vi "Main.vi"() -> ()   [LabVIEW 2010]
uses:
  <vilib>/Instr/_visa.llb/VISA Set IO Buffer Mask.ctl
  <vilib>/Instr/_visa.llb/VISA Flush IO Buffer Mask.ctl
  GlobalVar.vi
  <vilib>/Instr/_visa.llb/VISA Configure Serial Port (Instr).vi
panel:
  out "Frequency":dbl
  out "Enum":T1(ring)
  out "error":errorcluster
  out "error Connexion":errorcluster
  out "Stop main loop":bool
  in  "stop":bool
  in  "Tab Control":T2(tab)
  out "Comm_LEDTest":bool
  out "Comm_Reception":string caption="Reception"
  in  "Comm_TestConnection":bool
  in  "Comm_BaudRate":u32=9600 caption="Baud rate"
  in  "Comm_PortComm":refnum<visa-resource-name>="COM7" caption="Communication Port"
  in  "timeout (10sec)":u32=10000
  in  "Con_RefreshIntensity":bool caption="Bouton OK 12"
  in  "Con_RefreshRightTorque":bool caption="Bouton OK 12"
  out "Con_XYIntensity":cluster{"Y":dbl[], "Y":dbl[]}[](graph) caption="Intensity"
  out "Con_XYRightTorque":cluster{"Y":dbl[], "Y":dbl[]}[](graph) caption="Motor right Torque"
  in  "Con_RefreshLeftTorque":bool caption="Bouton OK 12"
  out "Con_XYLeftTorque":cluster{"Y":dbl[], "Y":dbl[]}[](graph) caption="Motor left Torque"
  out "Con_IntensityMax":bool caption="Max Intensity"
  in  "Con_Intensity":string[][](array[string]) caption="Intensity (A)"
  in  "Con_MotorRightTorque":string[][](array[string]) caption="Motor right Torque (N.m)"
  out "Con_MotorLeftTorque":string[][](array[string]) caption="Motor left Torque (N.m)"
  in  "Ana_RefreshBattery":bool caption="Bouton OK 12"
  out "Ana_XYBattery":cluster{"Y":dbl[], "Y":dbl[]}[](graph) caption="Motor left Torque"
  in  "Ana_RefreshHandlebar":bool caption="Bouton OK 12"
  out "Ana_XYHandlebar":cluster{"Y":dbl[], "Y":dbl[]}[](graph) caption="Motor left Torque"
  out "Ana_Battery":string[][](array[string]) caption="Battery"
  out "Ana_Handlebar":string[][](array[string]) caption="Handlebar"
  in  "Inc_RefreshAcceleration":bool caption="Bouton OK 12"
  out "Ana_XYHandlebar 4":cluster{"Y":dbl[], "Y":dbl[]}[](graph) caption="Motor left Torque"
  in  "Inc_RefreshVelocityRightMotor":bool caption="Bouton OK 12"
  out "Ana_XYHandlebar 3":cluster{"Y":dbl[], "Y":dbl[]}[](graph) caption="Motor left Torque"
  in  "Inc_RefreshVelocityLeftMotor":bool caption="Bouton OK 12"
  out "Ana_XYHandlebar 2":cluster{"Y":dbl[], "Y":dbl[]}[](graph) caption="Motor left Torque"
  out "Inc_Acceleration":string[][](array[string]) caption="Acceleration"
  out "Inc_VelocityRightMotor":string[][](array[string]) caption="Velocity Right motor"
  out "Inc_VelocityLeftMotor":string[][](array[string]) caption="Velocity left motor"
  out "Other_AngleOUT":string[][](array[string]) caption="Angle Out of range"
  out "Other_SpeedSaturation":string[][](array[string]) caption="Speed saturation"
  out "Other_Distance":string[][](array[string]) caption="Distance"
  out "Other_Angle":string[][](array[string]) caption="Angle"
  out "Spe_XY":cluster{dbl, dbl}[](graph) caption="XY Graph"
  in  "Spe_Time":dbl caption="Time"
  in  "Spe_SendAnalysis":bool caption="Send Analysis"
  in  "Spe_Frequency":dbl caption="Frequency"
  in  "Spe_Liste":string(combo) caption="Type"
  in  "Config_VelocitySaturation":dbl caption="VelocitySaturation"
  in  "Config_Sendvelocitysaturation":bool caption="Set velocity saturation"
  out "Config_Ready":string caption="Ready"
  out "Config_CurrentState":string caption="Current state"
  in  "Config_SendReady":bool caption="Ready ?"
  in  "Config_SendCurrentState":bool caption="Current state ?"
  in  "Config_SendRestart":bool caption="Re Start system"
  in  "Config_SendSTOP":bool caption="STOP system"
  out "Config_tCoefKalman":dbl caption="tCoef Kalman"
  in  "Config_ReceiveKalman":bool
  in  "Config_SendCoefKalman":bool
  in  "Config_CoefKalman":dbl caption="Coef Kalman"
  in  "Config_SendCoefAcc":bool
  in  "Config_CoefAcc":dbl caption="Coef System Acc"
  out "Config_Coefdir":dbl caption="tCoef direction"
  in  "Config_SendCoefDir":bool
  in  "Coef DIR":dbl
  in  "Config_ReceiveCoefDir":bool
  out "Config_tD":dbl caption="tD"
  out "Config_tI":dbl caption="tI"
  out "Config_tK":dbl caption="tK"
  in  "Config_ReceiveD":bool caption="Bouton OK 6"
  in  "Config_ReceiveI":bool
  in  "Config_ReceiveK":bool
  in  "Config_SendD":bool
  in  "Config_SendI":bool
  in  "Config_SendK":bool
  in  "Config_D":dbl caption="D"
  in  "Config_I":dbl caption="I"
  in  "Config_K":dbl caption="K"
  in  "Config_SendPID":bool
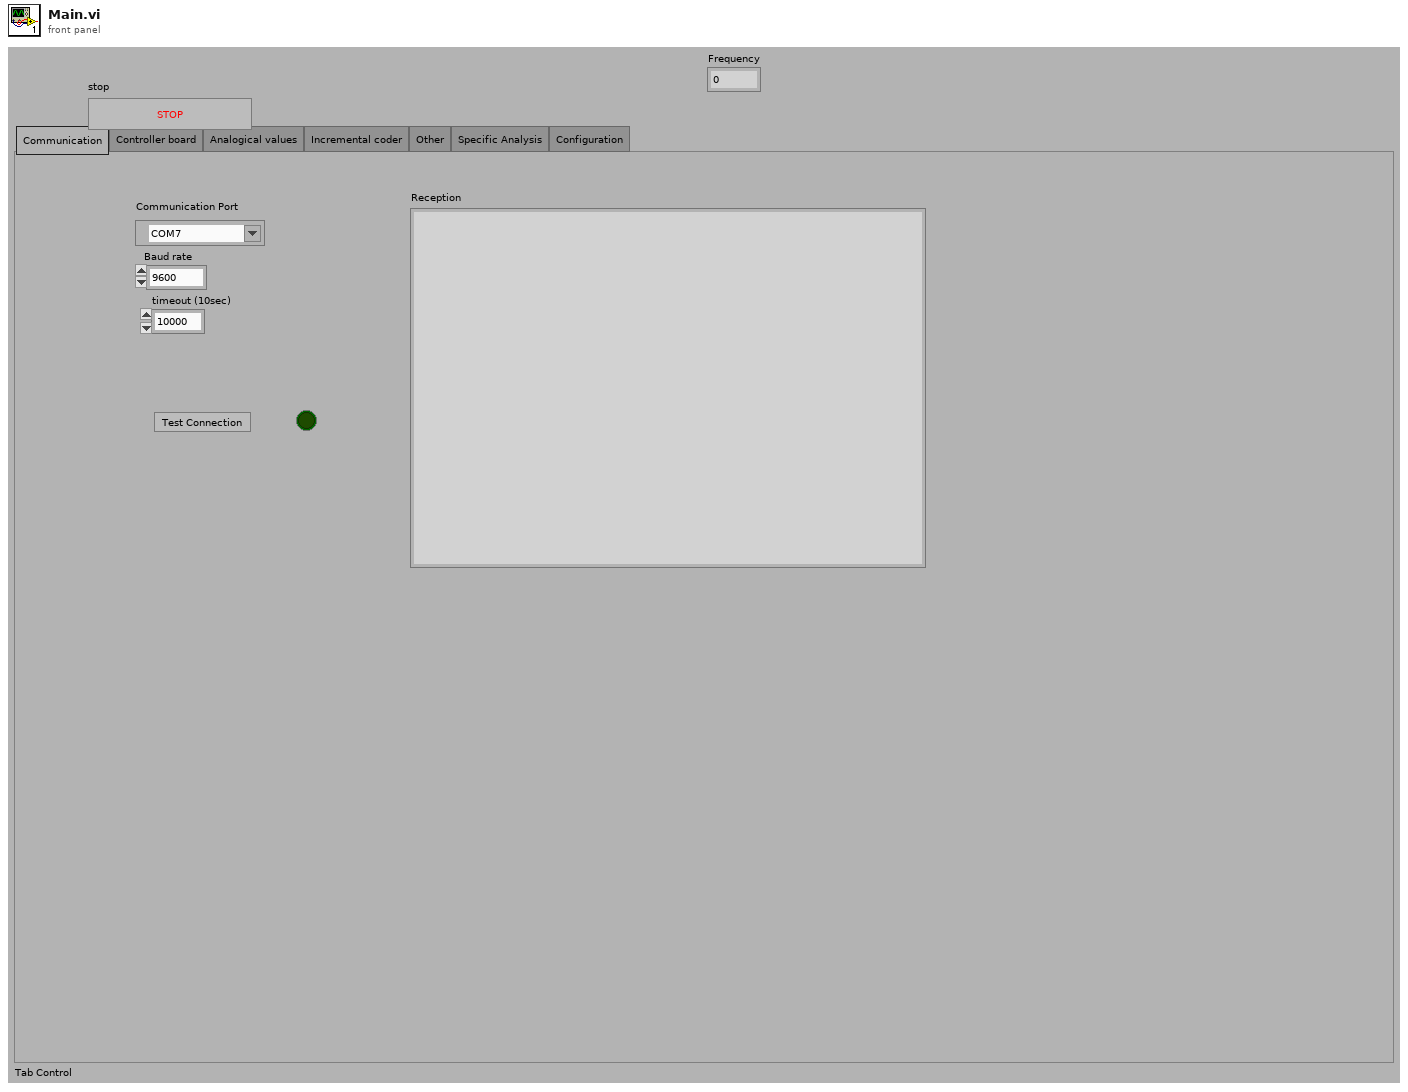
[diagram p1: front panel]
types:
  T1 = enum16{"SendAnalysis", "TestConnection", "Waiting"}
  T2 = enum32{"Communication", "Controller board", "Analogical values", "Incremental coder", "Other", "Specific Analysis", "Configuration"}
  T3 = typedef "VISA Set IO Buffer Mask.ctl" = u16
  T4 = typedef "VISA Flush IO Buffer Mask.ctl" = u16
  T5 = enum8{"Enabled", "Disabled", "Disabled and Grayed Out"}
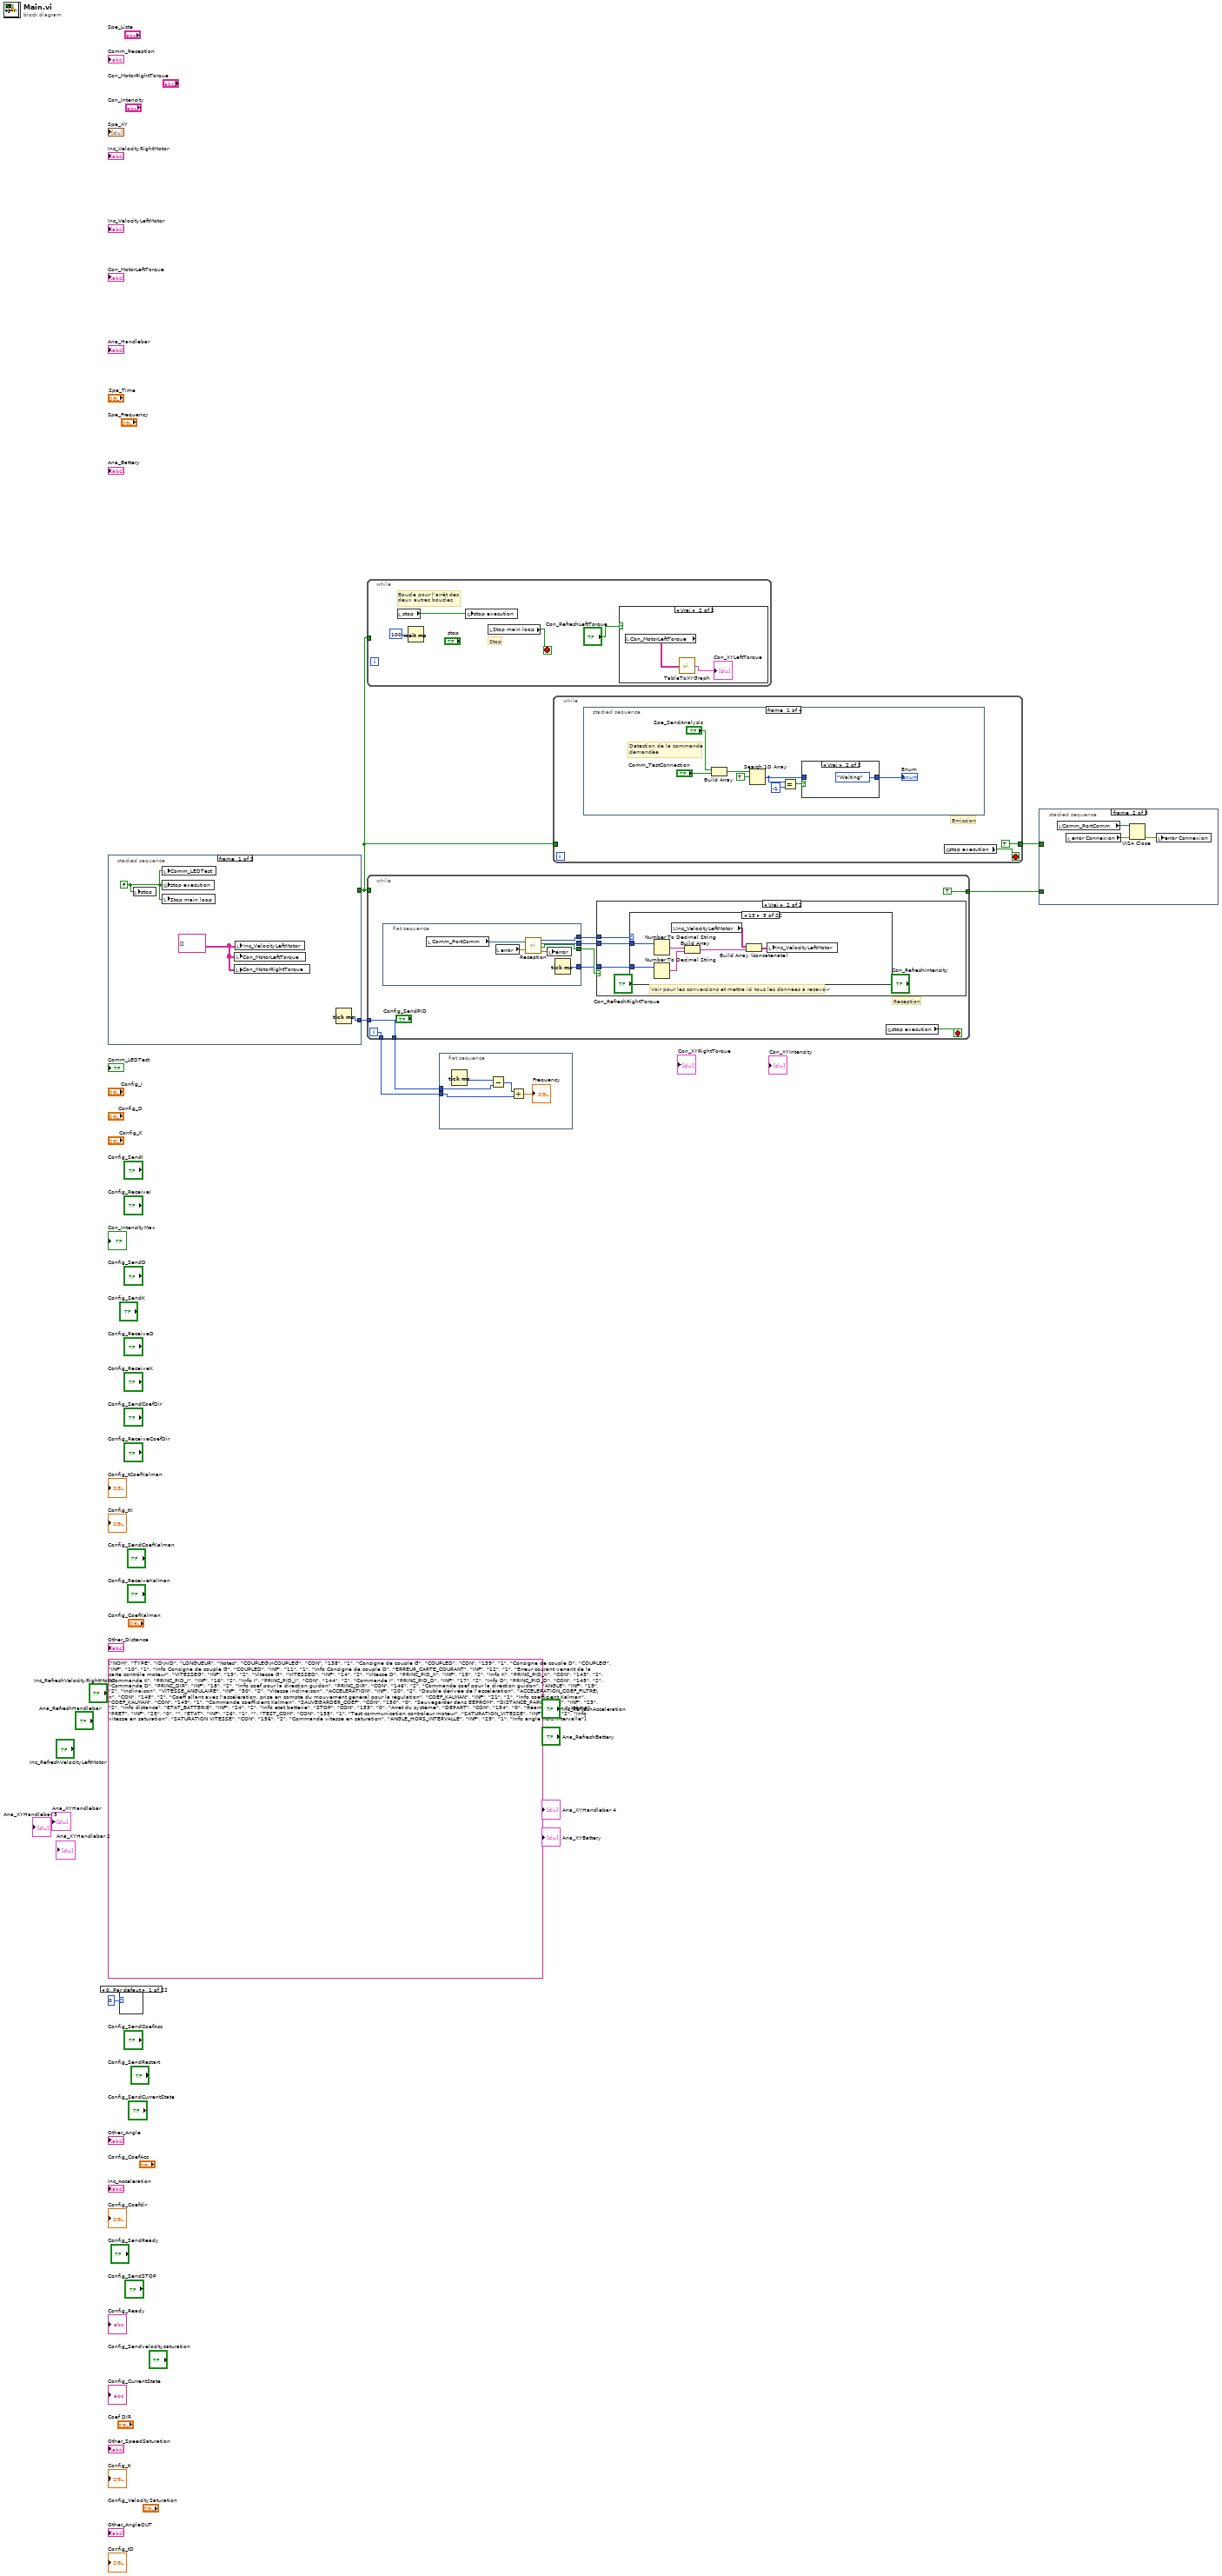
[diagram p0: block diagram]
diagram:
  (unwired) string[][] [["NOM", "TYPE", "ID\nID", "LONGUEUR", "Notes"], ["COUPLEG\nCOUPLEG", "CON", "138", "1", "Consigne de couple G"], ["COUPLED", "CON", "139", "1", "Consigne de couple D"], ["COUPLEG", "INF", "10", "1", "Info Consigne de couple G"], ["COUPLED", "INF", "11", "1", "Info Consigne de couple D"], ["ERREUR_CARTE_COURANT", "INF", "12", "1", "Erreur courant venant de la carte contrôle moteur"], ["VITESSEG", "INF", "13", "2", "Vitesse G"], ["VITESSED", "INF", "14", "2", "Vitesse D"], ["PRINC_PID_K", "INF", "15", "2", "Info K"], ["PRINC_PID_K", "CON", "143", "2", "Commande K"], ["PRINC_PID_I", "INF", "16", "2", "Info I"], ["PRINC_PID_I", "CON", "144", "2", "Commande I"], ["PRINC_PID_D", "INF", "17", "2", "Info D"], ["PRINC_PID_D", "CON", "145", "2", "Commande D"], ["PRINC_DIR", "INF", "18", "2", "Info coef pour la direction guidon"], ["PRINC_DIR", "CON", "146", "2", "Commande coef pour la direction guidon"], ["ANGLE", "INF", "19", "2", "Inclinaison"], ["VITESSE_ANGULAIRE", "INF", "30", "2", "Vitesse inclinaison"], ["ACCELERATION", "INF", "20", "2", "Double dérivée de l'accélération"], ["ACCELERATION_COEF_FILTRE\n", "CON", "148", "2", "Coeff allant avec l'accélération, prise en compte du mouvement général pour la régulation"], ["COEF_KALMAN", "INF", "21", "1", "Info coefficient Kalman"], ["COEF_KALMAN", "CON", "149", "1", "Commande coefficient Kalman"], ["SAUVEGARDER_COEF", "CON", "150", "0", "Sauvegarder dans EEPROM"], ["DISTANCE_PARCOURUE", "INF", "23", "2", "Info distance"], ["ETAT_BATTERIE", "INF", "24", "2", "Info etat batterie"], ["STOP", "CON", "153", "0", "Arret du système"], ["DEPART", "CON", "154", "0", "Réarmage du système"], ["PRET", "INF", "25", "0", ""], ["ETAT", "INF", "26", "1", ""], ["TEST_COM", "CON", "155", "1", "Test communication controleur moteur"], ["SATURATION_VITESSE", "INF", "28", "2", "Info vitesse en saturation"], ["SATURATION VITESSE", "CON", "156", "2", "Commande vitesse en saturation"], ["ANGLE_HORS_INTERVALLE", "INF", "29", "1", "Info angle hors intervalle"]]
  n1 = stacked-sequence {
    tunnel: [_ _ TRUE] -> w7
    tunnel: [w8 _ _] -> w3
    frame #0 {
      w9 = string[][] [] ("Velocity motor left")
      w10 = FALSE ("Comm_LEDTest")
      n2 = local write "stop"(w10) -> ()
      n3 = local write "Comm_LEDTest"(w10) -> ()
      n4 = global write "GlobalVar.vi" "stop execution"(w10) -> ()
      n5 = local write "Stop main loop"(w10) -> ()
      n6 = local write "Con_MotorLeftTorque"(w9) -> ()
      n7 = local write "Con_MotorRightTorque"(w9) -> ()
      n8 = local write "Inc_VelocityLeftMotor"(w9) -> ()
      n9 = Tick Count (ms)() -> (millisecond timer value=w8:u32)
    }
    frame #1 {
      w12 = T3 48 items=["Buffer d'entrées (E/S)"=16, "Buffer de sorties (E/S)"=32, "Buffer d'entrées et de sorties (E/S)"=48] ("Mask")
      w16 = T4 16 items=["Vider le buffer d'entrées"=16, "Écrire le buffer de sorties sur le périphérique"=32, "Vider le buffer d'entrées (Pas d'E/S)"=64, "Vider le buffer de sorties"=128] ("Mask")
      w20 = u16 0 items=["None"=0, "XON/XOFF"=1, "RTS/CTS"=2, "DTR/DSR"=4] ("flow control")
      w21 = u16 10 items=["1.0"=10, "1.5"=15, "2.0"=20] ("stop bits")
      w23 = u16 0 items=["None", "Odd", "Even", "Mark", "Space"] ("parity")
      # "Initial"
      n10 = local write "Tab Control"(T2."Communication" ("Tab Control")) -> ()
      n11 = call-poly "VISA Configure Serial Port"("VISA resource name"="Comm_PortComm", "timeout (10sec)"="timeout (10sec)", "baud rate (9600)"="Comm_BaudRate", "data bits (8)"=u16 8 ("data bits"), "parity (0:none)"=w23, "stop bits (10: 1 bit)"=w21, "flow control (0:none)"=w20) -> ("VISA resource name out"=w17:refnum<visa-resource-name>, "error out"=w14:errorcluster)  [unwired: 2 in, 5 out]
      "error Connexion" <- w14
      "error" <- w14
      n12 = VISA Set I/O Buffer Size(VISA resource name=w17, mask (16)=w12, size (4096)=u32 524288 ("taille (4096)"), error in (no error)=w14) -> (VISA resource name out=w15:refnum<visa-resource-name>, error out=w13:errorcluster)
      n13 = VISA Flush I/O Buffer(VISA resource name=w15, mask (16)=w16, error in (no error)=w13) -> ()  [unwired: 2 out]
    }
    frame #2 {
      # "OK Initialisation"
    }
  }
  n14 = case shown="0, Par défaut" 0 {
    frame 0, Default {
    }
    frame 10 {
    }
    frame 11 {
    }
    frame 12 {
    }
    frame 13 {
    }
    frame 14 {
    }
    frame 15 {
    }
    frame 16 {
    }
    frame 17 {
    }
    frame 18 {
    }
    frame 19 {
    }
    frame 20 {
    }
    frame 21 {
    }
    frame 22 {
    }
    frame 23 {
    }
    frame 24 {
    }
    frame 25 {
    }
    frame 26 {
    }
    frame 27 {
    }
    frame 28 {
    }
    frame 29 {
    }
    frame 30 {
    }
  }
  n15 = while {
    tunnel: w7 -> [_]
    stop <- w29 stop-if-true
    # "Boucle pour l'arrêt des \ndeux autres boucles"
    # "Stop"
    n16 = local read "stop"() -> (w30:bool)
    n17 = Wait (ms)(milliseconds to wait=u32 100) -> ()  [unwired: 1 out]
    n18 = global write "GlobalVar.vi" "stop execution"(w30) -> ()
    n19 = local read "Stop main loop"() -> (w29:bool)
    n20 = case shown="Vrai" "Con_RefreshLeftTorque" {
      frame False {
      }
      frame True {
        n21 = local read "Con_MotorLeftTorque"() -> (w31:string[][])
        n22 = call "TableToXYGraph.vi"("Input Table"=w31) -> ("XY Graph"=→"Con_XYLeftTorque":cluster{"Y":dbl[], "Y":dbl[]}[])
      }
    }
  }
  n23 = while {
    tunnel: w7 -> [_]
    tunnel: [TRUE] -> w6
    tunnel: w3 -> [w33]
    tunnel: [w34] -> w2
    tunnel: [w33] -> w1
    i -> [w34]
    stop <- w39 stop-if-true
    # "Reception"
    n24 = flat-sequence {
      tunnel: [w45] -> w38
      tunnel: [w44] -> w37
      tunnel: [w43] -> w36
      tunnel: [w42] -> w35
      frame #0 {
        n25 = local read "Comm_PortComm"() -> (w47:refnum<visa-resource-name>)
        n26 = local read "error"() -> (w46:errorcluster)
        n27 = call "Reception.vi"("entrée d'erreur (pas d'erreur)"=w46, "Nom de ressource VISA"=w47) -> ("Sortie d'erreur"=w41:errorcluster, "Checksum OK?"=w45:bool, "Data"=w43:i32, "ID byte"=w44:i32)
        n28 = local write "error"(w41) -> ()
        n29 = Tick Count (ms)() -> (millisecond timer value=w42:u32)
      }
    }
    n30 = case shown="Vrai" w38 {
      tunnel: w37 -> [_ w50]
      tunnel: w36 -> [_ w49]
      tunnel: w35 -> [_ w48]
      frame False {
      }
      frame True {
        # "Voir pour les conversions et mettre ici tous les données à recevoir"
        n31 = case shown="13" w50 {
          tunnel: w49 -> [_ w56 w59 _ w65 _ _ _ _ _ _ _ _ _ _ _ _ _ _ _ _ _]
          tunnel: w48 -> [_ w55 w58 _ w66 _ _ _ _ _ _ _ _ _ _ _ _ _ _ _ _ _]
          frame 0, Default {
          }
          frame 10 {
            n32 = Number To Decimal String(number=w56) -> (decimal integer string=w54:string)  [unwired: 1 in]
            n33 = Number To Decimal String(number=w55) -> (decimal integer string=w53:string)  [unwired: 1 in]
            n34 = Build Array(w54, w53) -> (w52:string[])
            n35 = local read "Con_MotorLeftTorque"() -> (w57:string[][])
            n36 = Build Array (concatenate)(w57, w52) -> (w51:string[][])
            n37 = local write "Con_MotorLeftTorque"(w51) -> ()
          }
          frame 11 {
            n38 = Number To Decimal String(number=w59) -> (decimal integer string=w63:string)  [unwired: 1 in]
            n39 = Number To Decimal String(number=w58) -> (decimal integer string=w62:string)  [unwired: 1 in]
            n40 = Build Array(w63, w62) -> (w61:string[])
            n41 = local read "Con_MotorRightTorque"() -> (w64:string[][])
            n42 = Build Array (concatenate)(w64, w61) -> (w60:string[][])
            n43 = local write "Con_MotorRightTorque"(w60) -> ()
          }
          frame 12 {
          }
          frame 13 {
            n44 = Number To Decimal String(number=w65) -> (decimal integer string=w70:string)  [unwired: 1 in]
            n45 = Number To Decimal String(number=w66) -> (decimal integer string=w69:string)  [unwired: 1 in]
            n46 = local read "Inc_VelocityLeftMotor"() -> (w71:string[][])
            n47 = Build Array(w70, w69) -> (w68:string[])
            n48 = Build Array (concatenate)(w71, w68) -> (w67:string[][])
            n49 = local write "Inc_VelocityLeftMotor"(w67) -> ()
          }
          frame 14 {
          }
          frame 15 {
          }
          frame 16 {
          }
          frame 17 {
          }
          frame 18 {
          }
          frame 19 {
          }
          frame 20 {
          }
          frame 21 {
          }
          frame 22 {
          }
          frame 23 {
          }
          frame 24 {
          }
          frame 25 {
          }
          frame 26 {
          }
          frame 27 {
          }
          frame 28 {
          }
          frame 29 {
          }
          frame 30 {
          }
        }
      }
    }
    n50 = global read "GlobalVar.vi" "stop execution"() -> (w39:bool)
  }
  n51 = flat-sequence {
    tunnel: w2 -> [w73]
    tunnel: w1 -> [w75]
    frame #0 {
      n52 = Tick Count (ms)() -> (millisecond timer value=w76:u32)
      n53 = Subtract(x=w76, y=w75) -> (x-y=w74:u32)
      n54 = Divide(x=w74, y=w73) -> (x/y=→"Frequency":dbl)
    }
  }
  n55 = while {
    tunnel: w7 -> [_]
    tunnel: [TRUE] -> w5
    stop <- w77 stop-if-true
    # "Emission"
    n56 = stacked-sequence {
      frame #0 {
        # "Detection de la commande\ndemandée"
        n57 = Build Array("Spe_SendAnalysis", "Comm_TestConnection") -> (w84:bool[])
        n58 = Search 1D Array(1D array=w84, element=TRUE) -> (index of element=w79:i32)  [unwired: 1 in]
        n59 = Equal?(x=w79, y=-1) -> (x = y?=w81:bool)
        n60 = case shown="Vrai" w81 {
          tunnel: [w87 T1."Waiting" ("Enum 2")] -> w80
          tunnel: w79 -> [w87 _]
          frame False {
          }
          frame True {
          }
        }
        "Enum" <- w80
      }
      frame #1 {
        n61 = local read "Enum"() -> (w90:T1)
        n62 = Not Equal?(x=w90, y=T1."Waiting") -> (x != y?=w91:bool)
        n63 = case shown="Vrai" w91 {
          frame False {
          }
          frame True {
            w92 = T5."Disabled and Grayed Out" ("Disabled")
            # "Disable all commands"
            n64 = property on="Spe_SendAnalysis" class="Bool"("DisabledEnum"=w92) -> ()  [unwired: 2 in, 2 out]
            n65 = property on="Comm_TestConnection" class="Bool"("DisabledEnum"=w92) -> ()  [unwired: 2 in, 2 out]
          }
        }
      }
      frame #2 {
        # "Traitement de la commande,\nboucles pour des mesures avec création \nde la trame série,\nautre pour la configuration"
        n66 = Wait (ms)(milliseconds to wait=u32 500) -> ()  [unwired: 1 out]
      }
      frame #3 {
        w94 = T5."Enabled" ("Disabled")
        # "Disable all commands"
        # "Activate all commands"
        n67 = property on="Spe_SendAnalysis" class="Bool"("DisabledEnum"=w94) -> ()  [unwired: 2 in, 2 out]
        n68 = property on="Comm_TestConnection" class="Bool"("DisabledEnum"=w94) -> ()  [unwired: 2 in, 2 out]
      }
    }
    n69 = global read "GlobalVar.vi" "stop execution"() -> (w77:bool)
  }
  n70 = stacked-sequence {
    tunnel: w6 -> [_ _ _]
    tunnel: w5 -> [w95 _ _]
    frame #0 {
      # "Finalisation"
      "Stop main loop" <- w95
    }
    frame #1 {
      n71 = local read "Comm_PortComm"() -> (w98:refnum<visa-resource-name>)
      n72 = local read "error Connexion"() -> (w97:errorcluster)
      n73 = VISA Close(VISA resource name=w98, error in (no error)=w97) -> (error out=w96:errorcluster)
      n74 = local write "error Connexion"(w96) -> ()
    }
    frame #2 {
      n75 = local read "error Connexion"() -> (w101:errorcluster)
      n76 = local read "error"() -> (w100:errorcluster)
      n77 = Merge Errors(w100, w101) -> (w99:errorcluster)
      n78 = call <vilib>:"Simple Error Handler.vi"("error in (no error)"=w99) -> ()  [unwired: 4 in, 5 out]
    }
  }
